vi "MYRIO.vi"() -> ()   [LabVIEW 2016]
doc: "Demonstrates the use of User Datagram Protocol (UDP) to receive data from the host computer."
uses:
  <vilib>/myRIO/Instrument Drivers/Onboard IO/DIO/typedefs/DIO Reference.ctl
  <vilib>/myRIO/Common/Instrument Driver Framework/Utilities/typedefs/myRIO Generic Hardware Reference.ctl
  <vilib>/myRIO/Common/Instrument Driver Framework/Utilities/typedefs/Hardware Version Enum.ctl
  <vilib>/myRIO/Common/Instrument Driver Framework/Utilities/typedefs/myRIO v1.0 Reference.ctl
  <vilib>/myRIO/Common/Instrument Driver Framework/Utilities/typedefs/Generic FPGA Reference.ctl
  <vilib>/myRIO/Common/Instrument Driver Framework/myRIO v1.0/DIO/typedefs/DIO Channels List.ctl
  <vilib>/myRIO/Common/Instrument Driver Framework/myRIO v1.0/DIO/typedefs/DIO Channels Enum.ctl
  <vilib>/userdefined/High Color/nirio_resource_hc.ctl
  <vilib>/myRIO/Common/Instrument Driver Framework/Utilities/vis/Is FPGA Ref Available.vi
  <vilib>/myRIO/Common/Instrument Driver Framework/myRIO v1.0/DIO/vis/myRIO v1.1 Open DIO.vi
  <vilib>/myRIO/Instrument Drivers/Onboard IO/DIO/vis/Write.vi
  <vilib>/myRIO/Common/Instrument Driver Framework/Utilities/vis/Validate Channels.vi
  <vilib>/myRIO/Common/Instrument Driver Framework/myRIO v1.0/DIO/vis/myRIO v1.0 Reserve DIO.vi
  <vilib>/myRIO/Common/Instrument Driver Framework/myRIO v1.0/UART/vis/myRIO v1.0 Close UART.vi
  <vilib>/myRIO/Common/Instrument Driver Framework/myRIO v1.0/Resource Manager/vis/myRIO v1.0 Reserve Channel List.vi
  <vilib>/myRIO/Common/Instrument Driver Framework/myRIO v1.0/DIO/vis/myRIO v1.0 Build MUX Configuration DIO.vi
  <vilib>/myRIO/Common/Instrument Driver Framework/myRIO v1.0/Resource Manager/vis/myRIO v1.0 Reserve Channel.vi
  <vilib>/myRIO/Common/Instrument Driver Framework/myRIO v1.0/Resource Manager/vis/myRIO v1.0 Unreserve Channel.vi
  <vilib>/myRIO/Common/Instrument Driver Framework/myRIO v1.0/Resource Manager/vis/myRIO v1.0 Create Configuration List.vi
  <vilib>/myRIO/Common/Instrument Driver Framework/myRIO v1.0/Resource Manager/vis/myRIO v1.0 Build Mutex Name.vi
  <vilib>/Utility/VariantDataType/GetNumericInfo.vi
  <vilib>/Utility/error.llb/Error Cluster From Error Code.vi
  <vilib>/myRIO/Common/Instrument Driver Framework/myRIO v1.0/myRIO v1.1 Open.vi
  <vilib>/myRIO/Common/Instrument Driver Framework/Utilities/vis/IO Manager.vi
  <vilib>/myRIO/Common/Instrument Driver Framework/Utilities/vis/Configuration Manager.vi
  <vilib>/myRIO/Common/Instrument Driver Framework/myRIO v1.0/Resource Manager/vis/myRIO v1.0 Configure IO.vi
  <vilib>/myRIO/Common/Instrument Driver Framework/myRIO v1.0/myRIO v1.0 Close.vi
  <vilib>/myRIO/Common/Instrument Driver Framework/myRIO v1.0/DIO/vis/myRIO v1.0 Write DIO.vi
  <vilib>/myRIO/Common/Instrument Driver Framework/Utilities/vis/FPGA Ref Manager.vi
  <vilib>/myRIO/Common/Instrument Driver Framework/myRIO v1.0/myRIO v1.0 Reset FPGA.vi
  <vilib>/myRIO/Common/Instrument Driver Framework/myRIO v1.0/IRQ/vis/myRIO v1.0 IRQ Info FGV.vi
  <vilib>/myRIO/Common/Instrument Driver Framework/myRIO v1.0/IRQ/vis/myRIO v1.0 Timer IRQ Info FGV.vi
  <vilib>/myRIO/Common/Instrument Driver Framework/myRIO v1.0/IRQ/vis/myRIO v1.0 ISR Agent.vi
  <vilib>/myRIO/Express VI/Onboard IO/DO/DO Express VI.xnode
  <vilib>/myRIO/Instrument Drivers/Onboard IO/DIO/vis/myRIO DIO Open.xnode
  <vilib>/myRIO/Express VI/Onboard Devices/LED/LED Express VI.xnode
  <vilib>/myRIO/Instrument Drivers/Onboard IO/DIO/DIO.lvlib
  <vilib>/myRIO/Instrument Drivers/Utilities/Utilities.lvlib
panel:
  out "etapa 1":bool
  out "LED Status":bool[](array[boolean])
  out "error out":errorcluster
  in  "Stop":bool
  # "Overview: Demonstrates the use of User Datagram Protocol (UDP) to receive data from the host computer.\nInstructions:\n1. Ensure Desktop Main.vi is already running.\n2. Run this VI.\n3. Observe the LEDs on the myRIO device and the value of LED Status on this VI. They change when the value of LED on Desktop Main.vi changes.\n4. Click Stop to stop this VI."
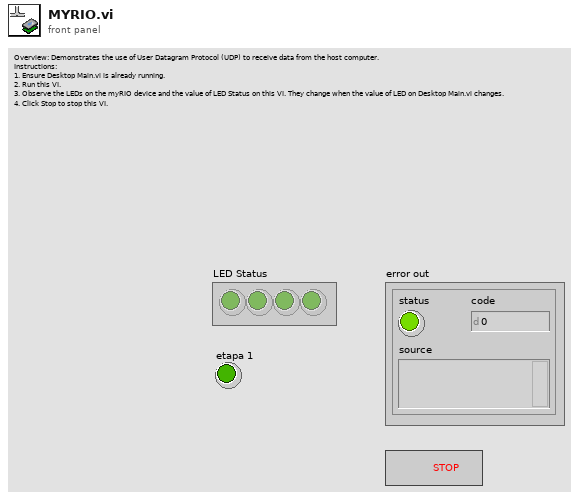
[diagram p1: front panel]
types:
  T1 = typedef "DIO.lvlib/DIO Reference.ctl" = cluster{"myRIO Reference":T2, "DIO Channels List":T6}
  T2 = typedef "myRIO Generic Hardware Reference.ctl" = cluster{"myRIO Model":T3, "myRIO Hardware Reference":T4}
  T3 = typedef "Hardware Version Enum.ctl" = enum16{"Unknown", "myRIO-1900", "myRIO-1950", "roboRIO", "NI ELVIS RIO CM"}
  T4 = typedef "myRIO v1.0 Reference.ctl" = cluster{"Generic FPGA Reference":T5, "Allow multiple opens":bool}
  T5 = typedef "Generic FPGA Reference.ctl" = refnum<k20>
  T6 = typedef "DIO Channels List.ctl" = T7[]
  T7 = typedef "DIO Channels Enum.ctl" = enum16{"Not Connected", "C/DIO0", "C/DIO1", "C/DIO2", "C/DIO3", "C/DIO4", "C/DIO5", "C/DIO6", "C/DIO7", "A/DIO0", "A/DIO1", "A/DIO2", "A/DIO3", "A/DIO4", "A/DIO5", "A/DIO6", "A/DIO7", "A/DIO8", "A/DIO9", "A/DIO10", "A/DIO11", "A/DIO12", "A/DIO13", "A/DIO14", "A/DIO15", "B/DIO0", "B/DIO1", "B/DIO2", "B/DIO3", "B/DIO4", "B/DIO5", "B/DIO6", "B/DIO7", "B/DIO8", "B/DIO9", "B/DIO10", "B/DIO11", "B/DIO12", "B/DIO13", "B/DIO14", "B/DIO15", "LED0", "LED1", "LED2", "LED3", "Button0", "DIO/DIO0", "DIO/DIO1", "DIO/DIO2", "DIO/DIO3", "DIO/DIO4", "DIO/DIO5", "DIO/DIO6", "DIO/DIO7", "DIO/DIO8", "DIO/DIO9", "SPI/CS0", "SPI/CS1", "SPI/CS2", "SPI/CS3", "LED RADIO (Green)", "LED RADIO (Red)", "LED COMM (Green)", "LED COMM (Red)", "LED MODE (Green)", "LED MODE (Red)"}
  T8 = typedef "nirio_resource_hc.ctl" = tag
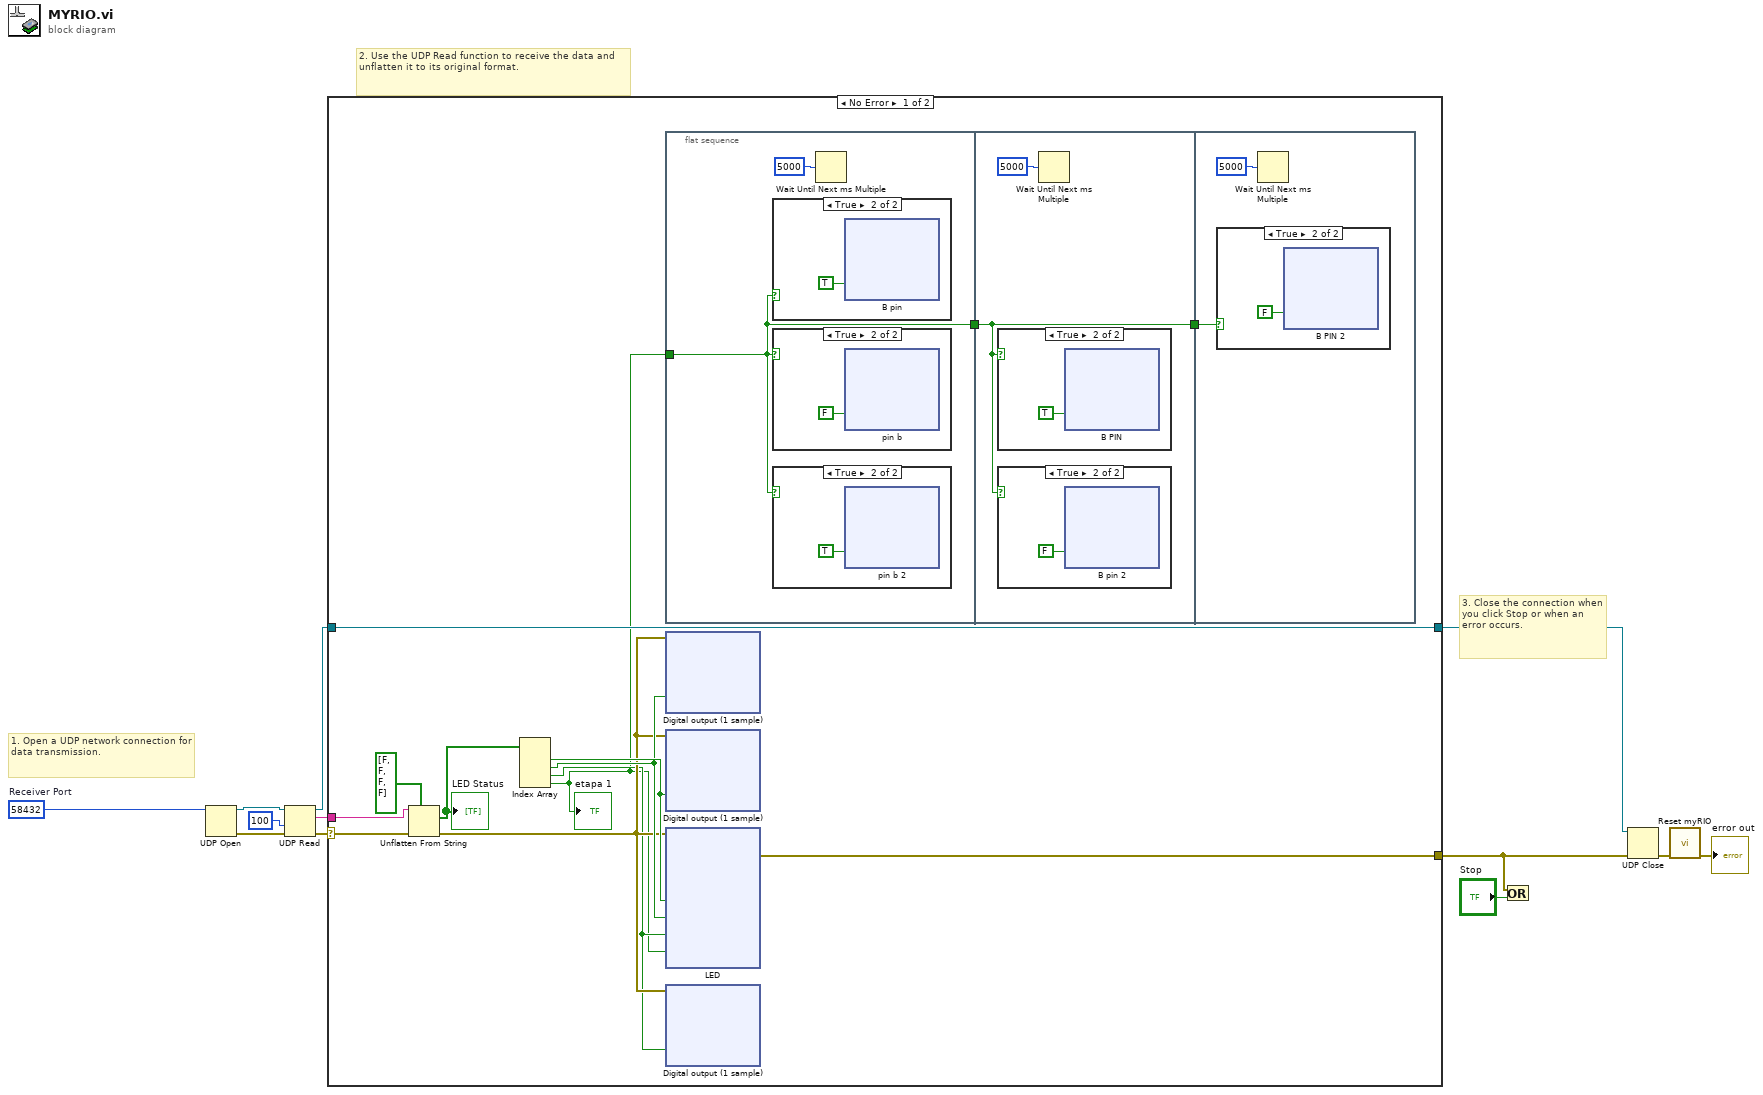
[diagram p0: block diagram]
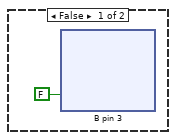
[diagram p2: hidden frame]
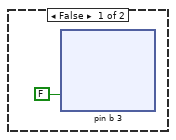
[diagram p3: hidden frame]
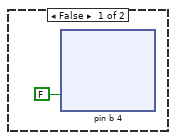
[diagram p4: hidden frame]
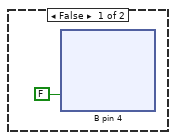
[diagram p5: hidden frame]
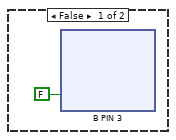
[diagram p6: hidden frame]
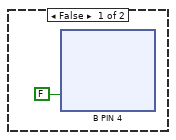
[diagram p7: hidden frame]
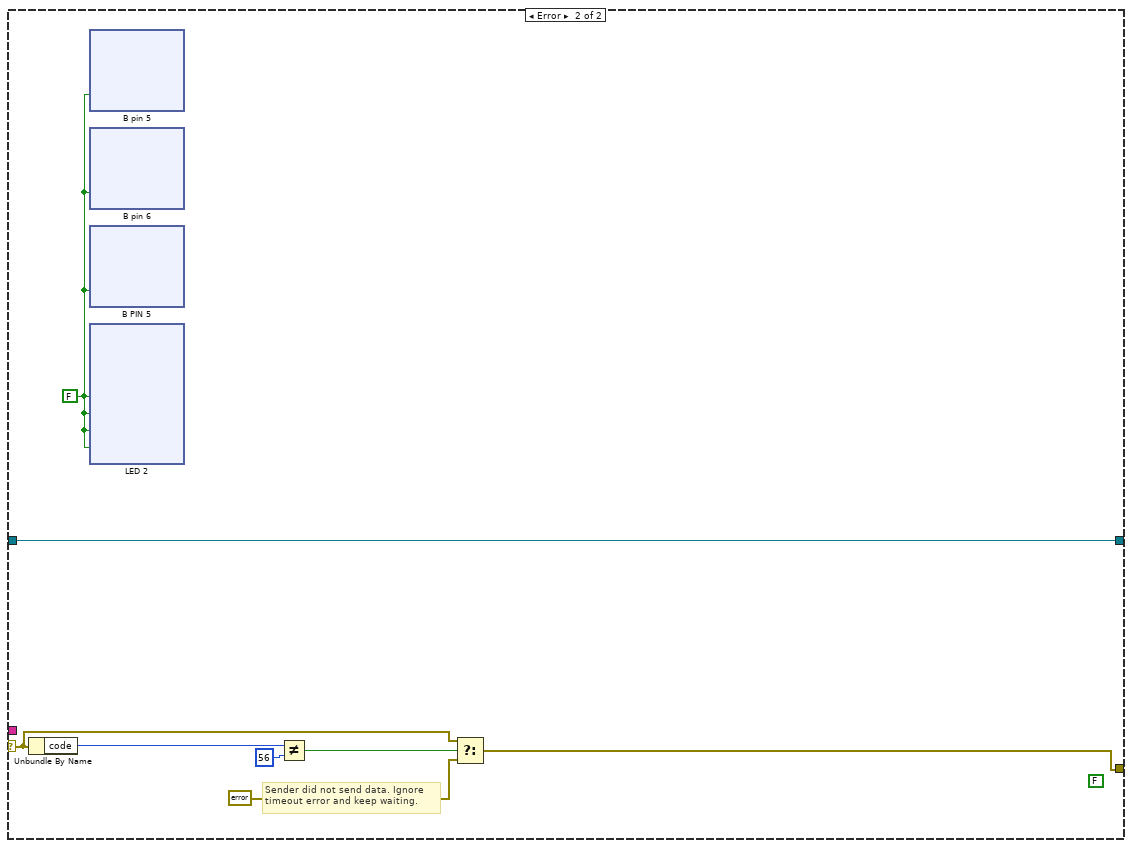
[diagram p8: hidden frame]
diagram:
  w8 = u16 58432  # Receiver Port
  # "2. Use the UDP Read function to receive the data and unflatten it to its original format."
  # "3. Close the connection when you click Stop or when an error occurs."
  # "1. Open a UDP network connection for data transmission."
  n1 = UDP Open(11:w8) -> (port=w12:refnum<k16>, 0:w11:errorcluster)  [unwired: 4 in, 1 out]
  n2 = UDP Read(connection ID=w12, timeout ms (25000)=100, 8:w11) -> (data out=w1:string, error out=w3:errorcluster, 3:w4:refnum<k16>)  [unwired: 1 in, 2 out]
  n3 = case shown="No Error" w3 {
    selector: w3 -> [w22 w609]
    tunnel: [w20 w608] -> w9
    tunnel: w4 -> [w23 w614]
    tunnel: [w23 w614] -> w10
    tunnel: w1 -> [w21 _]
    frame No Error {
      n4 = Unflatten From String(type=bool[] [FALSE, FALSE, FALSE, FALSE] ("LED Status"), binary string=w21, error in (no error)=w22) -> (value=w24:bool[], error out=w17:errorcluster)  [unwired: 2 in, 1 out]
      "LED Status" <- w24
      n5 = Index Array(array=w24) -> (element #1=w19:bool, element #2=w18:bool, element #3=w16:bool, element #4=w14:bool)  [unwired: 4 in]
      "etapa 1" <- w14
      n6 = flat-sequence {
        tunnel: [w26] -> w15
        tunnel: w14 -> [w26]
        tunnel: [w245] -> w13
        tunnel: w15 -> [w245]
        tunnel: w13 -> [w391]
        frame #0 {
          n7 = case shown="True" w26 {
            frame False {
              n8 = xnode "B pin 3"("B/DIO1 (Pin 13)"=FALSE) -> ()  [unwired: 1 in, 1 out]
            }
            frame True {
              n9 = xnode "B pin"("B/DIO1 (Pin 13)"=TRUE) -> ()  [unwired: 1 in, 1 out]
            }
          }
          n10 = case shown="True" w26 {
            frame False {
              n11 = xnode "pin b 4"("B/DIO0 (Pin 11)"=FALSE) -> ()  [unwired: 1 in, 1 out]
            }
            frame True {
              n12 = xnode "pin b"("B/DIO0 (Pin 11)"=FALSE) -> ()  [unwired: 1 in, 1 out]
            }
          }
          n13 = case shown="True" w26 {
            frame False {
              n14 = xnode "pin b 3"("B/DIO0 (Pin 11)"=FALSE) -> ()  [unwired: 1 in, 1 out]
            }
            frame True {
              n15 = xnode "pin b 2"("B/DIO0 (Pin 11)"=TRUE) -> ()  [unwired: 1 in, 1 out]
            }
          }
          n16 = Wait Until Next ms Multiple(millisecond multiple=u32 5000) -> ()  [unwired: 1 out]
        }
        frame #1 {
          n17 = case shown="True" w245 {
            frame False {
              n18 = xnode "B PIN 3"("B/DIO15 (Pin 34)"=FALSE ("B/DIO1 (Pin 13)")) -> ()  [unwired: 1 in, 1 out]
            }
            frame True {
              n19 = xnode "B PIN"("B/DIO15 (Pin 34)"=TRUE ("B/DIO1 (Pin 13)")) -> ()  [unwired: 1 in, 1 out]
            }
          }
          n20 = case shown="True" w245 {
            frame False {
              n21 = xnode "B pin 4"("B/DIO1 (Pin 13)"=FALSE) -> ()  [unwired: 1 in, 1 out]
            }
            frame True {
              n22 = xnode "B pin 2"("B/DIO1 (Pin 13)"=FALSE) -> ()  [unwired: 1 in, 1 out]
            }
          }
          n23 = Wait Until Next ms Multiple(millisecond multiple=u32 5000) -> ()  [unwired: 1 out]
        }
        frame #2 {
          n24 = case shown="True" w391 {
            frame False {
              n25 = xnode "B PIN 4"("B/DIO15 (Pin 34)"=FALSE ("B/DIO1 (Pin 13)")) -> ()  [unwired: 1 in, 1 out]
            }
            frame True {
              n26 = xnode "B PIN 2"("B/DIO15 (Pin 34)"=FALSE ("B/DIO1 (Pin 13)")) -> ()  [unwired: 1 in, 1 out]
            }
          }
          n27 = Wait Until Next ms Multiple(millisecond multiple=u32 5000) -> ()  [unwired: 1 out]
        }
      }
      n28 = xnode "Digital output (1 sample)"("B/DIO1 (Pin 13)"=w18, "error in (no error)"=w17) -> ()  [unwired: 1 out]
      n29 = xnode "Digital output (1 sample)"("B/DIO0 (Pin 11)"=w19, "error in (no error)"=w17) -> ()  [unwired: 1 out]
      n30 = xnode "LED"("LED0"=w19, "LED1"=w18, "LED2"=w16, "LED3"=w14, "error in (no error)"=w17) -> ("error out"=w20:errorcluster)
      n31 = xnode "Digital output (1 sample)"("B/DIO15 (Pin 34)"=w16, "error in (no error)"=w17) -> ()  [unwired: 1 out]
    }
    frame Error {
      w607 = FALSE
      (unwired) FALSE
      # "Sender did not send data. Ignore \ntimeout error and keep waiting."
      n32 = Unbundle By Name(w609) -> ("code"=w611:i32)
      n33 = xnode "B pin 5"("B/DIO1 (Pin 13)"=w607) -> ()  [unwired: 1 in, 1 out]
      n34 = xnode "B pin 6"("B/DIO0 (Pin 11)"=w607) -> ()  [unwired: 1 in, 1 out]
      n35 = xnode "B PIN 5"("B/DIO15 (Pin 34)"=w607) -> ()  [unwired: 1 in, 1 out]
      n36 = xnode "LED 2"("LED0"=w607, "LED1"=w607, "LED2"=w607, "LED3"=w607) -> ()  [unwired: 1 in, 1 out]
      n37 = Not Equal?(x=w611, y=56) -> (x != y?=w610:bool)
      n38 = Select(t=w609, s=w610, f=errorcluster {"status"=FALSE, "code"=0, "source"=""} ("error out")) -> (s? t:f=w608:errorcluster)
    }
  }
  n39 = Or(x=w9, y="Stop") -> ()  [unwired: 1 out]
  n40 = UDP Close(connection ID=w10, 8:w9) -> (error out=w7:errorcluster)  [unwired: 1 out]
  n41 = call <vilib>:"Reset myRIO.vi"("error in (no error)"=w7) -> ("error out"=→"error out":errorcluster)  [unwired: 10 in]
